vi "CryoConnect.vi"() -> (0 "connection ID":refnum<k5>)   [LabVIEW 2019]
panel:
  in  "Address":string="localhost"
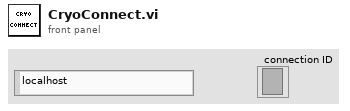
[diagram p1: front panel]
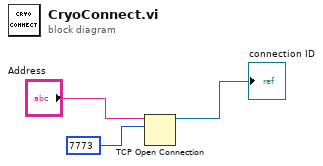
[diagram p0: block diagram]
diagram:
  n1 = TCP Open Connection(address="Address", remote port or service name=u16 7773) -> (connection ID=→"connection ID":refnum<k5>)  [unwired: 3 in, 1 out]
